vi "Clear Triggers.vi"(8 "error in (no error)":errorcluster, 11 "Camera in":refnum<class "Camera.lvclass">) -> (0 "error out":errorcluster, 3 "Camera":refnum<class "Camera.lvclass">)   [LabVIEW 2020, in "Camera.lvclass"]
uses:
  Camera.lvclass
  Camera.lvclass/Camera.ctl
  bin/gindustrialcam_32-1.dll
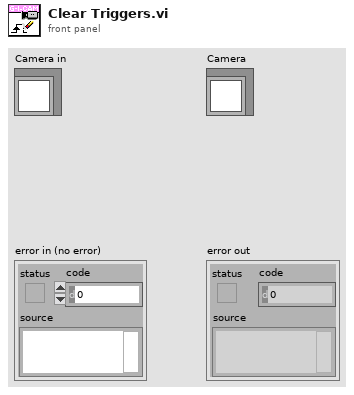
[diagram p1: front panel]
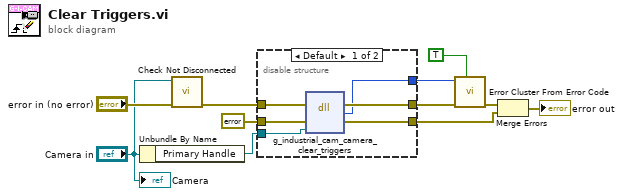
[diagram p0: block diagram]
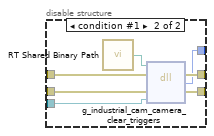
[diagram p2: hidden frame]
diagram:
  n1 = Unbundle By Name("Camera in") -> ("Primary Handle"=w3:refnum<data-value>)
  n2 = call "Check Not Disconnected.vi"("error in (no error)"="error in (no error)", "Camera in"="Camera in") -> ("error out"=w2:errorcluster)  [unwired: 9 in]
  n3 = disable-structure shown="Default" {
    disable-tunnel: [w17 w24] -> w9
    disable-tunnel: [w16 w23] -> w8
    disable-tunnel: [w15 w22] -> w6
    disable-tunnel: errorcluster {"status"=FALSE, "code"=0, "source"=""} ("error constant") -> [w14 w21]
    disable-tunnel: w3 -> [w13 w20]
    disable-tunnel: w2 -> [w12 w19]
    frame condition #0 (active) {
      n4 = dll-call lib="C:/serenial/lib/g-industrial-camera/LabVIEW/g_industrial_cam/bin/gindustrialcam_*-1.*" fn="g_industrial_cam_camera_clear_triggers"(error in=w12, "err"=w14, "edvr"=w13) -> (error out=w17:errorcluster, "Mg_Error"=w16:i32, "err"=w15:errorcluster)  [unwired: 3 in, 1 out]
    }
    frame condition #1 {
      n5 = call "RT Shared Binary Path.vi"() -> ("Path"=w18:path)
      n6 = dll-call lib="C:/serenial/lib/g-industrial-camera/LabVIEW/g_industrial_cam/bin/gindustrialcam_*-1.*" fn="g_industrial_cam_camera_clear_triggers"(path in=w18, error in=w19, "err"=w21, "edvr"=w20) -> (error out=w24:errorcluster, "Mg_Error"=w23:i32, "err"=w22:errorcluster)  [unwired: 2 in, 1 out]
    }
  }
  n7 = call <vilib>:"Error Cluster From Error Code.vi"("show call chain? (False)"=TRUE, "error in (no error)"=w9, "error code (0)"=w8) -> ("error out"=w7:errorcluster)  [unwired: 6 in]
  n8 = Merge Errors(w7, w6) -> (→"error out":errorcluster)
  "Camera" <- "Camera in"
